vi "Get Ideal Fundamental and IMD Slopes UI.vi"(7 "OIP3":dbl, 9 "Target Pin Per Tone (dBm)":dbl, 10 "Target Pout Per Tone (dBm)":dbl, 11 "List of PINs":dbl[](array[numeric])) -> (1 "IMD Slope":dbl[](array[numeric]), 2 "Fundamental Slope":dbl[](array[numeric]), 3 "List of PINs":dbl[](array[numeric]), 5 "IIP3":dbl)   [LabVIEW 2023, in "FPT Intermodulation UI.lvlib"]
uses:
  <vilib>/Analysis/1siggen.llb/Ramp Pattern by Samples.vi
  FPT Intermodulation UI.lvlib
  <vilib>/Analysis/NI_AALBase.lvlib
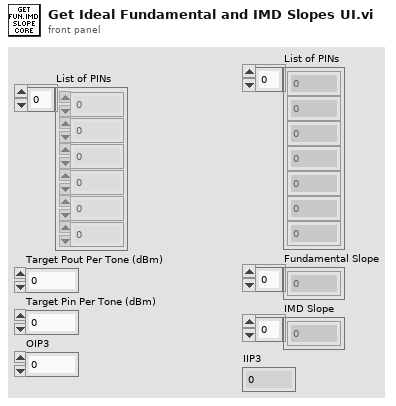
[diagram p1: front panel]
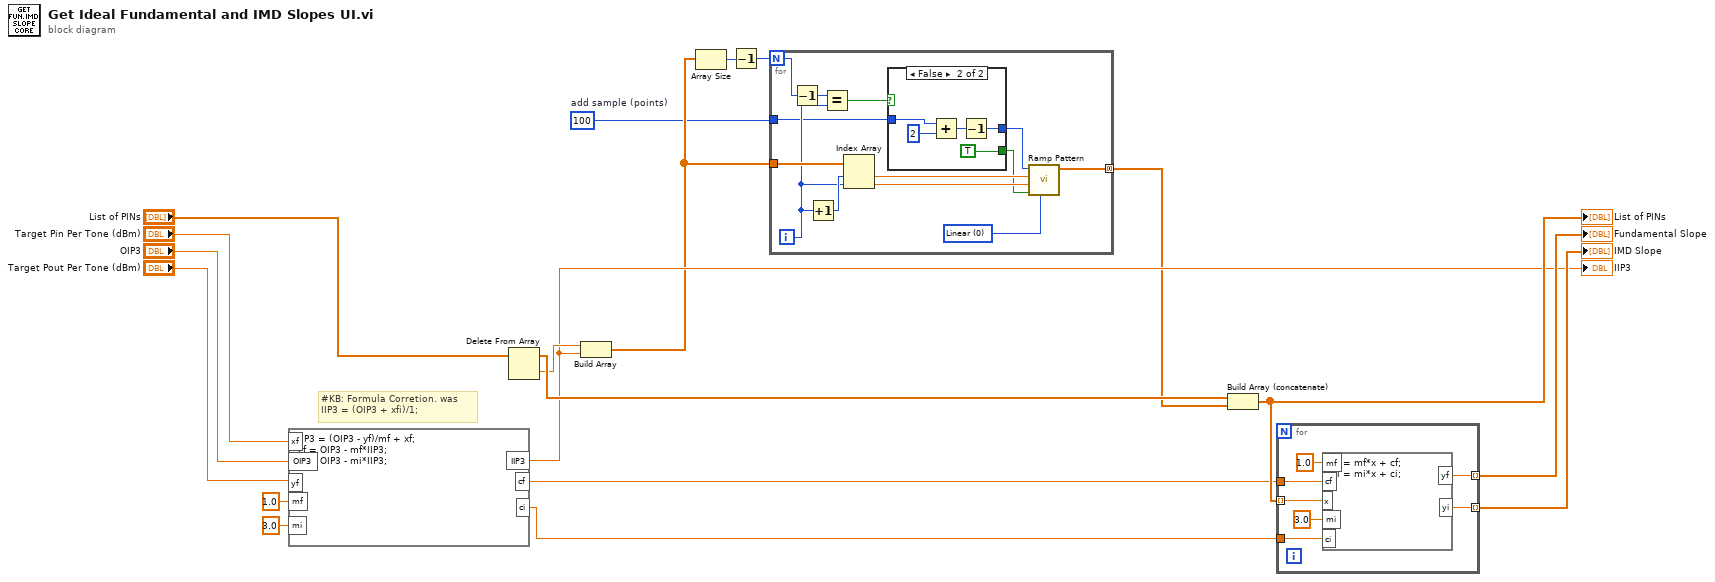
[diagram p0: block diagram]
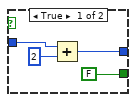
[diagram p2: hidden frame]
diagram:
  w2 = 100  # add sample (points)
  # "#KB: Formula Corretion. was \nIIP3 = (OIP3 + xfi)/1;"
  n1 = formula code="IIP3 = (OIP3 - yf)/mf + xf;\ncf = OIP3 - mf*IIP3;\nci = OIP3 - mi*IIP3;"("xf"="Target Pin Per Tone (dBm)", "OIP3"="OIP3", "yf"="Target Pout Per Tone (dBm)", "mf"=1.0 ("input variable"), "mi"=3.0 ("input variable")) -> ("IIP3"=w6:dbl, "cf"=w9:dbl, "ci"=w10:dbl)
  "IIP3" <- w6
  n2 = Delete From Array(array="List of PINs") -> (deleted portion=w15:dbl, array with subset deleted=w16:dbl[])  [unwired: 2 in]
  n3 = Build Array(w15, w6) -> (w3:dbl[])
  n4 = Array Size(array=w3) -> (size(s)=w4:i32)
  n5 = Decrement(x=w4) -> (x-1=w5:i32)
  n6 = for {
    N: w5 -> [w28]
    tunnel: w3 -> [w32]
    tunnel: [w26] -> w1 mode=concatenating
    tunnel: w2 -> [w21]
    i -> [w22]
    w20 = u16 0 items=["Linear", "Logarithmic"] ("type")
    n7 = Decrement(x=w28) -> (x-1=w27:i32)
    n8 = Increment(x=w22) -> (x+1=w31:i32)
    n9 = Equal?(x=w27, y=w22) -> (x = y?=w25:bool)
    n10 = Index Array(array=w32, index #1=w31, index #2=w22) -> (element #1=w30:dbl, element #2=w29:dbl)
    n11 = case shown="False" w25 {
      tunnel: [FALSE TRUE] -> w24
      tunnel: [w34 w38] -> w23
      tunnel: w21 -> [w33 w37]
      frame True {
        n12 = Add(x=w33, y=2) -> (x+y=w34:i32)
      }
      frame False {
        n13 = Add(x=w37, y=2) -> (x+y=w39:i32)
        n14 = Decrement(x=w39) -> (x-1=w38:i32)
      }
    }
    n15 = call-poly <vilib>:"Ramp Pattern.vi"("type"=w20, "exclude end?"=w24, "start"=w29, "end"=w30, "samples"=w23) -> ("Ramp Pattern"=w26:dbl[])  [unwired: 5 in, 1 out]
  }
  n16 = Build Array (concatenate)(w16, w1) -> (w18:dbl[])
  "List of PINs" <- w18
  n17 = for {
    tunnel: w18 -> [w44] mode=indexing
    tunnel: w9 -> [w46]
    tunnel: w10 -> [w45]
    tunnel: [w43] -> w11 mode=indexing
    tunnel: [w42] -> w12 mode=indexing
    n18 = formula code="yf = mf*x + cf;\nyi = mi*x + ci;"("mf"=1.0 ("input variable"), "x"=w44, "mi"=3.0 ("input variable"), "cf"=w46, "ci"=w45) -> ("yf"=w43:dbl, "yi"=w42:dbl)
  }
  "IMD Slope" <- w12
  "Fundamental Slope" <- w11
